vi "reboot.vi"(9 "id":u8, 10 "protocol_version":i32, 11 "port_num":i32) -> ()   [LabVIEW 2016, in "dxl_x86_c.lvlib"]
doc: "WINDECLSPEC void reboot (int port_num, int protocol_version, uint8_t id);"
uses:
  dxl_x86_c.lvlib
  dxl_x86_c.dll
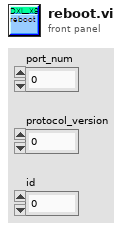
[diagram p1: front panel]
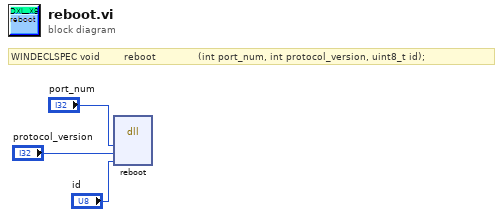
[diagram p0: block diagram]
diagram:
  # "WINDECLSPEC void        reboot              (int port_num, int protocol_version, uint8_t id);"
  n1 = dll-call lib="C:/Users/Platform/Desktop/DynamixelSDK/labview/dxl_x86_c.lvlib/dxl_x86_c.*" fn="reboot"("port_num"="port_num", "protocol_version"="protocol_version", "id"="id") -> ()  [unwired: 7 in, 2 out]
